vi "osa_init display.vi"(8 "error in (no error)":errorcluster, 9 "sensor LUT":variant, 10 "OSB status/control refnum in":refnum<vi>, 11 "display refnums in":T1) -> (0 "error out":errorcluster, 3 "display refnums out":T1)   [LabVIEW 2021]
panel:
  # "OSA subVI: init display, gray out OSB not mounted"
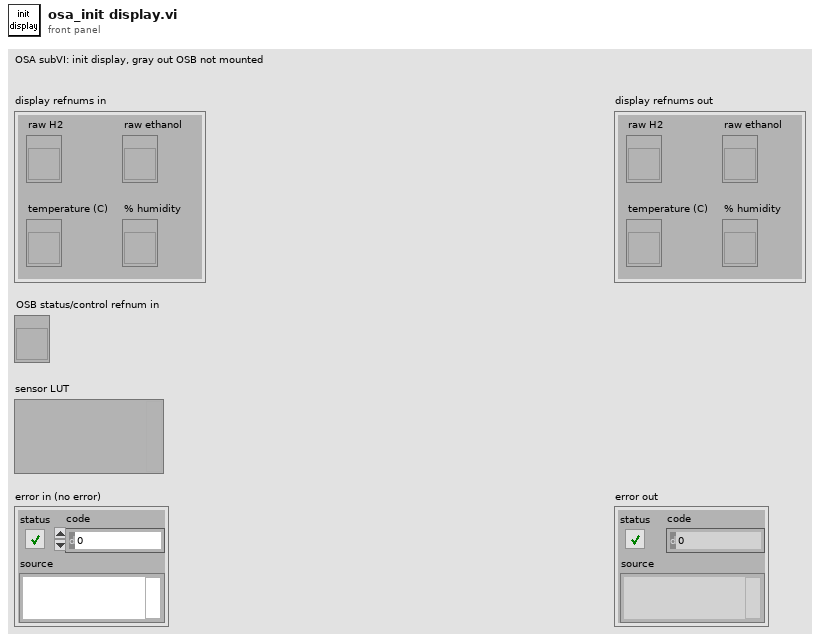
[diagram p1: front panel]
types:
  T1 = cluster{"raw H2":refnum<vi>, "raw ethanol":refnum<vi>, "temperature (C)":refnum<vi>, "% humidity":refnum<vi>}
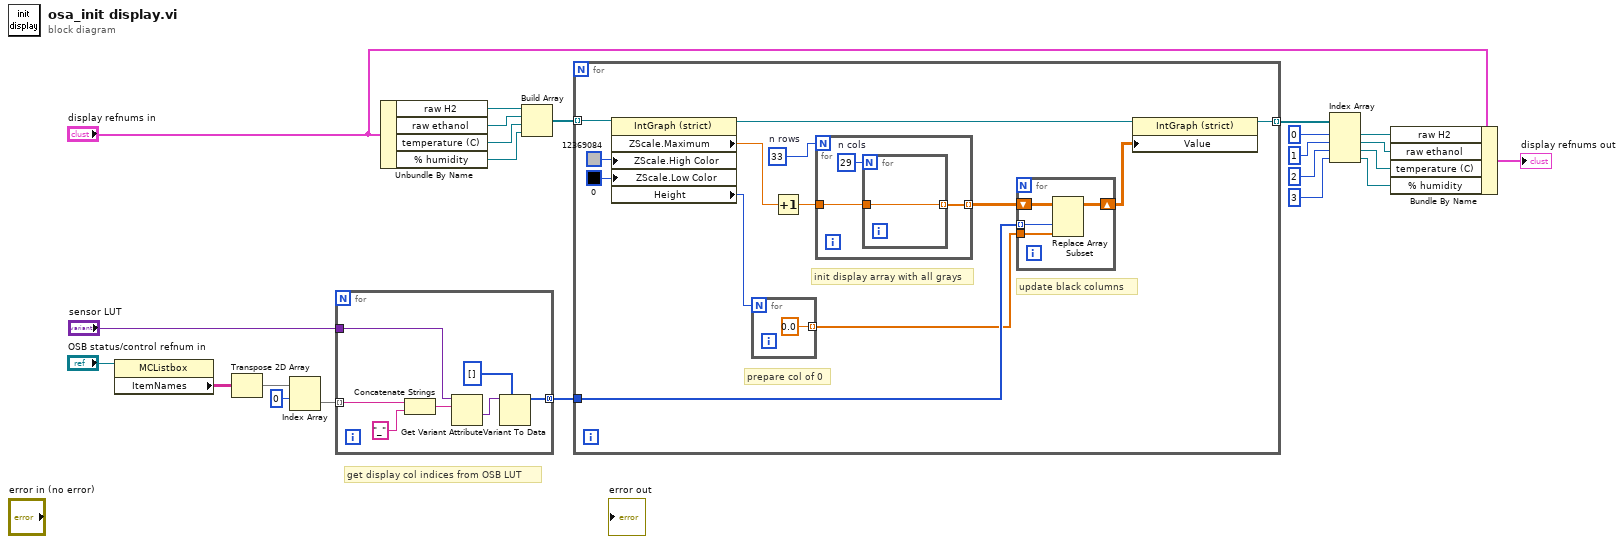
[diagram p0: block diagram]
diagram:
  # "get display col indices from OSB LUT"
  n1 = property class="MCListbox"(reference="OSB status/control refnum in") -> ("ItemNames"=w4:string[][])  [unwired: 1 in, 2 out]
  n2 = Transpose 2D Array(2D array=w4) -> (transposed array=w3:string[][])
  n3 = Index Array(array=w3, index (row)=0) -> (element=w1:string[])  [unwired: 1 in]
  n4 = for {
    tunnel: "sensor LUT" -> [w28]
    tunnel: [w25] -> w22 mode=concatenating
    tunnel: w1 -> [w24] mode=indexing
    n5 = Concatenate Strings(w24, "_") -> (w29:string)
    n6 = Get Variant Attribute(Variant=w28, name=w29) -> (value=w27:variant)  [unwired: 2 in, 3 out]
    n7 = Variant To Data(type=i32[] [], Variant=w27) -> (data=w25:i32[])  [unwired: 1 in, 1 out]
  }
  n8 = Unbundle By Name("display refnums in") -> ("raw H2"=w21:refnum<vi>, "raw ethanol"=w20:refnum<vi>, "temperature (C)"=w18:refnum<vi>, "% humidity"=w19:refnum<vi>)
  n9 = Build Array(w21, w20, w18, w19) -> (w17:refnum<vi>[])
  n10 = for {
    tunnel: w17 -> [w43] mode=indexing
    tunnel: w22 -> [w36]
    tunnel: [w31] -> w16 mode=indexing
    w40 = 33  # n rows
    # "update black columns"
    # "prepare col of 0"
    # "init display array with all grays"
    n11 = property class="IntGraph (strict)"(reference=w43, "ZScale.High Color"=u32 12369084, "ZScale.Low Color"=u32 0) -> (reference out=w32:refnum<vi>, "ZScale.Maximum"=w39:dbl, "Height"=w35:u32)  [unwired: 1 in, 1 out]
    n12 = for {
      N: w35 -> [_]
      tunnel: [0.0] -> w34 mode=indexing
    }
    n13 = Increment(x=w39) -> (x+1=w38:dbl)
    n14 = for {
      N: w40 -> [_]
      tunnel: w38 -> [w50]
      tunnel: [w49] -> w37 mode=indexing
      w51 = 29  # n cols
      n15 = for {
        N: w51 -> [_]
        tunnel: w50 -> [w52]
        tunnel: [w52] -> w49 mode=indexing
      }
    }
    n16 = for {
      shift-right: [w45] -> w33
      shift-left: w37 -> [w48]
      tunnel: w36 -> [w47] mode=indexing
      tunnel: w34 -> [w46]
      n17 = Replace Array Subset(array=w48, new element=w46, index (col)=w47) -> (w45:dbl[][])  [unwired: 1 in]
    }
    n18 = property class="IntGraph (strict)"(reference=w32, "Value"=w33) -> (reference out=w31:refnum<vi>)  [unwired: 1 in, 1 out]
  }
  n19 = Index Array(array=w16, index #1=0, index #2=1, index #3=2, index #4=3) -> (element #1=w11:refnum<vi>, element #2=w7:refnum<vi>, element #3=w8:refnum<vi>, element #4=w10:refnum<vi>)
  n20 = Bundle By Name(cluster="display refnums in", "raw H2"=w11, "raw ethanol"=w7, "temperature (C)"=w8, "% humidity"=w10) -> (→"display refnums out":T1)
